vi "8 swich.vi"() -> ()   [LabVIEW 2017]
panel:
  out "Numeric":i16
  in  "Boolean 11":bool
  in  "Boolean 10":bool
  in  "Boolean 9":bool
  in  "Boolean 8":bool
  in  "Boolean 7":bool
  in  "Boolean 6":bool
  in  "Boolean 5":bool
  in  "Boolean 4":bool
  in  "stop":bool
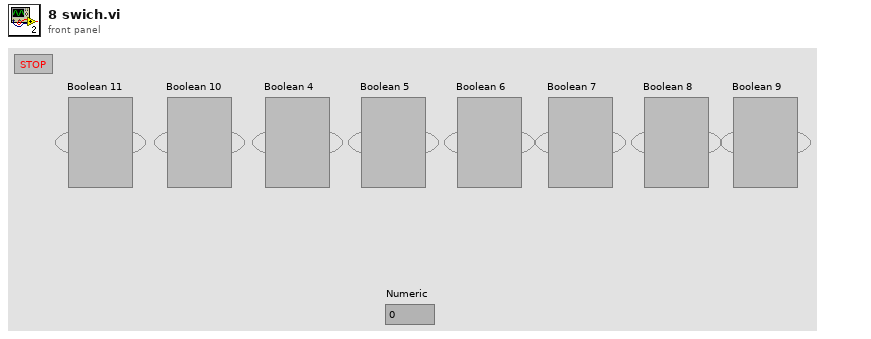
[diagram p1: front panel]
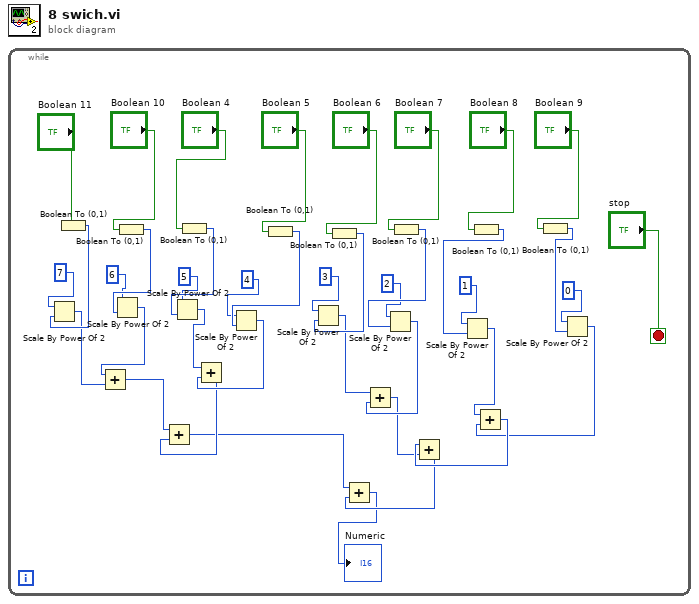
[diagram p0: block diagram]
diagram:
  n1 = while {
    stop <- "stop" stop-if-true
    n2 = Boolean To (0,1)(Boolean="Boolean 11") -> (0, 1=w16:i16)
    n3 = Scale By Power Of 2(n=7, x=w16) -> (x*2^n=w15:i16)
    n4 = Boolean To (0,1)(Boolean="Boolean 10") -> (0, 1=w37:i16)
    n5 = Scale By Power Of 2(n=6, x=w37) -> (x*2^n=w14:i16)
    n6 = Add(x=w14, y=w15) -> (x+y=w11:i16)
    n7 = Boolean To (0,1)(Boolean="Boolean 4") -> (0, 1=w34:i16)
    n8 = Scale By Power Of 2(n=5, x=w34) -> (x*2^n=w13:i16)
    n9 = Boolean To (0,1)(Boolean="Boolean 5") -> (0, 1=w31:i16)
    n10 = Scale By Power Of 2(n=4, x=w31) -> (x*2^n=w12:i16)
    n11 = Add(x=w13, y=w12) -> (x+y=w2:i16)
    n12 = Add(x=w11, y=w2) -> (x+y=w1:i16)
    n13 = Boolean To (0,1)(Boolean="Boolean 6") -> (0, 1=w27:i16)
    n14 = Scale By Power Of 2(n=3, x=w27) -> (x*2^n=w10:i16)
    n15 = Boolean To (0,1)(Boolean="Boolean 7") -> (0, 1=w25:i16)
    n16 = Scale By Power Of 2(n=2, x=w25) -> (x*2^n=w9:i16)
    n17 = Add(x=w10, y=w9) -> (x+y=w7:i16)
    n18 = Boolean To (0,1)(Boolean="Boolean 8") -> (0, 1=w22:i16)
    n19 = Scale By Power Of 2(n=1, x=w22) -> (x*2^n=w4:i16)
    n20 = Boolean To (0,1)(Boolean="Boolean 9") -> (0, 1=w18:i16)
    n21 = Scale By Power Of 2(n=0, x=w18) -> (x*2^n=w3:i16)
    n22 = Add(x=w4, y=w3) -> (x+y=w8:i16)
    n23 = Add(x=w8, y=w7) -> (x+y=w6:i16)
    n24 = Add(x=w1, y=w6) -> (x+y=→"Numeric":i16)
  }
